vi "Close References.vi"(7 "QRD":T1, 8 "error in":errorcluster) -> (0 "error out":errorcluster, 5 "QRD Out":T1)   [LabVIEW 2025]
uses:
  Controls/Queues-Refs-Data.ctl
  Builds/Queue Wrappers.lvlibp/Q Packet.ctl
  Builds/Queue Wrappers.lvlibp
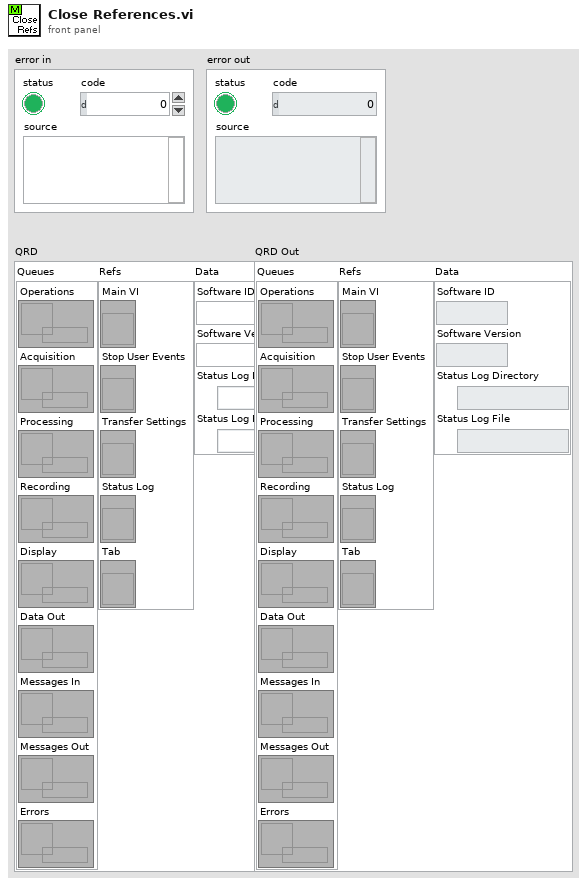
[diagram p1: front panel]
types:
  T1 = typedef "Queues-Refs-Data.ctl" = cluster{"Queues":cluster{"Operations":refnum<queue>, "Acquisition":refnum<queue>, "Processing":refnum<queue>, "Recording":refnum<queue>, "Display":refnum<queue>, "Data Out":refnum<queue>, "Messages In":refnum<queue>, "Messages Out":refnum<queue>, "Errors":refnum<queue>}, "Refs":cluster{"Main VI":refnum<vi>, "Stop User Events":refnum<vi>, "Transfer Settings":refnum<vi>, "Status Log":refnum<vi>, "Tab":refnum<vi>}, "Data":cluster{"Software ID":string, "Software Version":string, "Status Log Directory":path, "Status Log File":path}}
  T2 = cluster{"Main VI":refnum<vi>, "Stop User Events":refnum<vi>, "Transfer Settings":refnum<vi>, "Status Log":refnum<vi>, "Tab":refnum<vi>}
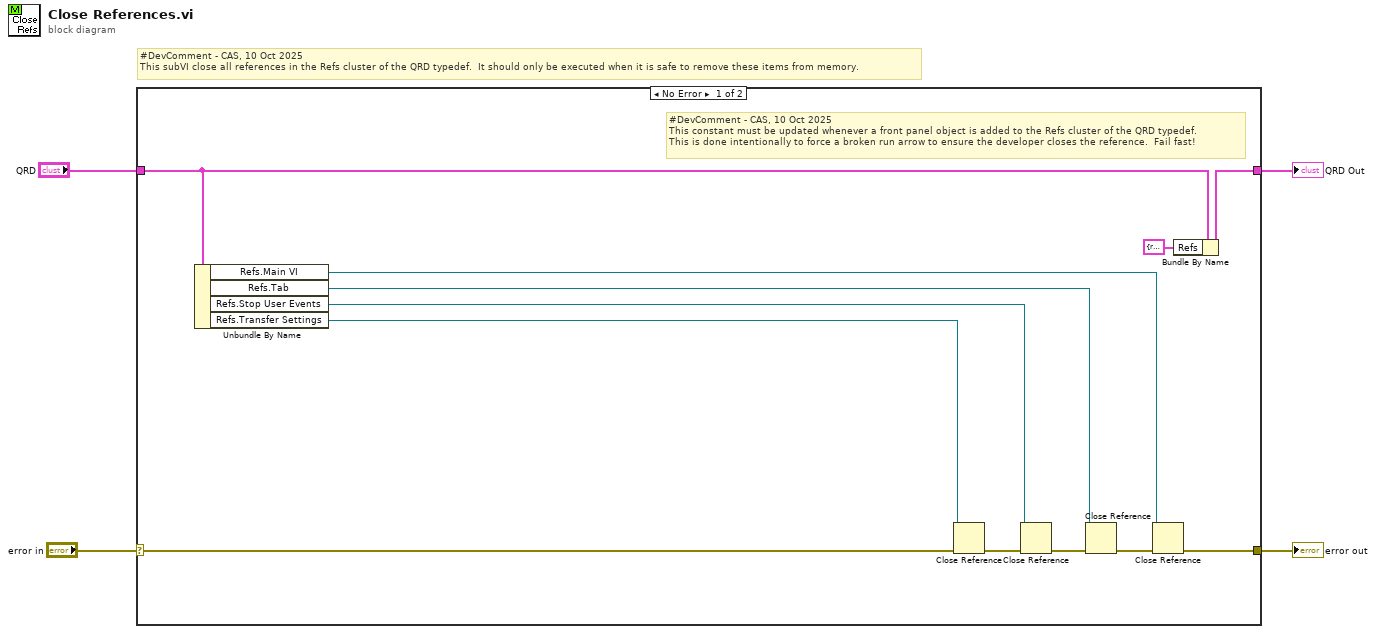
[diagram p0: block diagram]
diagram:
  # "#DevComment - CAS, 10 Oct 2025\nThis subVI close all references in the Refs cluster of the QRD typedef.  It should only be executed when it is safe to remove these items from memory."
  n1 = case shown="No Error" "error in" {
    selector: "error in" -> [w10 w17]
    tunnel: "QRD" -> [w15 w18]
    tunnel: [w16 w18] -> w2
    tunnel: [w12 w17] -> w1
    frame No Error {
      # "#DevComment - CAS, 10 Oct 2025\nThis constant must be updated whenever a front panel object is added to the Refs cluster of the QRD typedef.\nThis is done intentionally to force a broken run arrow to ensure the developer closes the reference.  Fail fast!"
      n2 = Unbundle By Name(w15) -> ("Refs.Main VI"=w13:refnum<vi>, "Refs.Tab"=w14:refnum<vi>, "Refs.Stop User Events"=w7:refnum<vi>, "Refs.Transfer Settings"=w6:refnum<vi>)
      n3 = Close Reference(reference=w6, error in (no error)=w10) -> (error out=w9:errorcluster)
      n4 = Close Reference(reference=w7, error in (no error)=w9) -> (error out=w8:errorcluster)
      n5 = Close Reference(reference=w14, error in (no error)=w8) -> (error out=w11:errorcluster)
      n6 = Close Reference(reference=w13, error in (no error)=w11) -> (error out=w12:errorcluster)
      n7 = Bundle By Name(cluster=w15, "Refs"=T2 {"Main VI"=refnum, "Stop User Events"=refnum, "Transfer Settings"=refnum, "Status Log"=refnum, "Tab"=refnum}) -> (w16:T1)
    }
    frame Error {
    }
  }
  "error out" <- w1
  "QRD Out" <- w2
